vi "GetQY_0.vi"(2 "error in":errorcluster) -> (0 "error out":errorcluster, 1 "data":string)   [LabVIEW 2010]
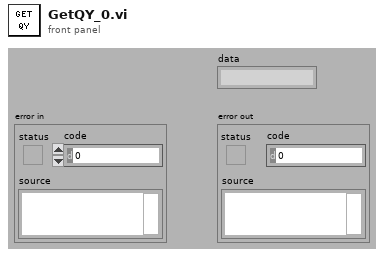
[diagram p1: front panel]
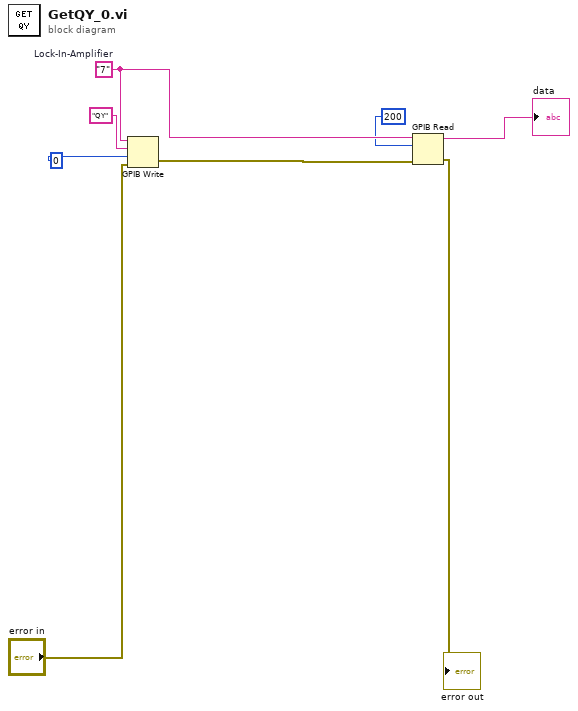
[diagram p0: block diagram]
diagram:
  w5 = "7"  # Lock-In-Amplifier
  n1 = GPIB Write(0:w5, 1:"QY", 2:i16 0 ("mode (0)"), 3:"error in") -> (6:w7:errorcluster)  [unwired: 1 in, 1 out]
  n2 = GPIB Read(0:w5, 1:200, 3:w7) -> (5:→"data":string, 7:→"error out":errorcluster)  [unwired: 2 in, 1 out]
